vi "TCP-Write (1D SGL).vi"(0 "connection ID":refnum<k5>, 5 "data":sgl[](array[numeric]), 9 "timeout (ms)":i32=5000, 11 "error in (no error)":errorcluster) -> (4 "connection ID out":refnum<k5>, 8 "bytes written":i32, 15 "error out":errorcluster)   [LabVIEW 2020]
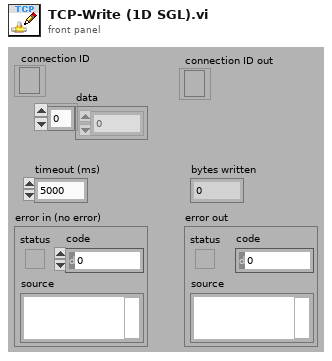
[diagram p1: front panel]
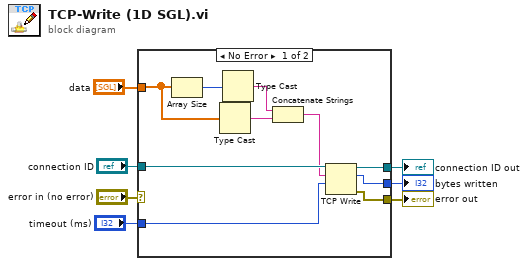
[diagram p0: block diagram]
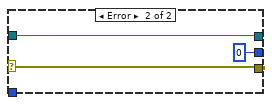
[diagram p2: hidden frame]
diagram:
  n1 = case shown="No Error" "error in (no error)" {
    selector: "error in (no error)" -> [_ w19]
    tunnel: [w9 w19] -> w1
    tunnel: [w17 w20] -> w7
    tunnel: "connection ID" -> [w13 w20]
    tunnel: "timeout (ms)" -> [w15 _]
    tunnel: [w14 0 ("bytes written")] -> w4
    tunnel: "data" -> [w8 _]
    frame No Error {
      n2 = Array Size(array=w8) -> (size(s)=w11:i32)
      n3 = Type Cast(x=w8) -> (*(type *) &x=w16:string)  [unwired: 1 in]
      n4 = Type Cast(x=w11) -> (*(type *) &x=w10:string)  [unwired: 1 in]
      n5 = Concatenate Strings(w10, w16) -> (w12:string)
      n6 = TCP Write(connection ID=w13, data in=w12, 9:w15) -> (connection ID out=w17:refnum<k5>, bytes written=w14:i32, error out=w9:errorcluster)  [unwired: 1 in]
    }
    frame Error {
    }
  }
  "error out" <- w1
  "bytes written" <- w4
  "connection ID out" <- w7
